vi "NonDuplicateArrays.vi"(8 "error in":errorcluster, 9 "string in":string, 11 "array in":string[](array[string])) -> (0 "error out":errorcluster, 3 "array out":string[](array[string]))   [LabVIEW 2023, in "CEF.lvlib"]
doc: "This Vi checks if the string exist in the array, if it doesnt it adds it to the array.Copyright 2017 National Instruments Corporation\n\nLicensed under the Apache License, Version 2.0 (the \"License\"); you may not use this file except in compliance with the License. You may obtain a copy of the License at http://www.apache.org/licenses/LICENSE-2.0\nUnless required by applicable law or agreed to in writing, software distributed under the License is distributed on an \"AS IS\" BASIS, WITHOUT WARRANTIES OR CONDITIONS OF ANY KIND, either express or implied. See the License for the specific language governing permissions and limitations under the License."
uses:
  CEF.lvlib
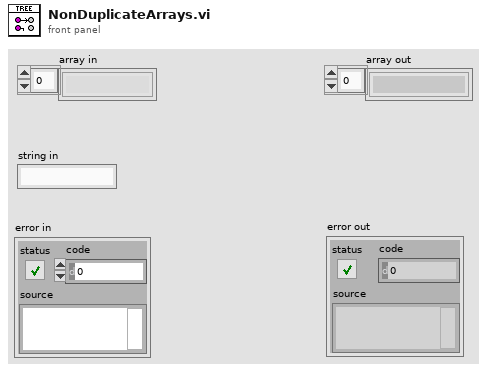
[diagram p1: front panel]
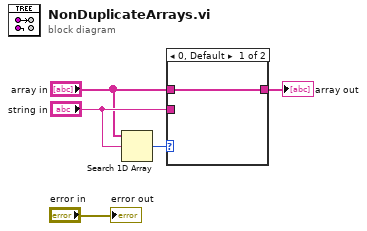
[diagram p0: block diagram]
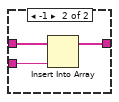
[diagram p2: hidden frame]
diagram:
  n1 = Search 1D Array(1D array="array in", element="string in") -> (index of element=w1:i32)  [unwired: 1 in]
  n2 = case shown="0, Default" w1 {
    tunnel: [w6 w8] -> w2
    tunnel: "array in" -> [w6 w9]
    tunnel: "string in" -> [_ w7]
    frame 0, Default {
    }
    frame -1 {
      n3 = Insert Into Array(array=w9, new element=w7) -> (w8:string[])  [unwired: 1 in]
    }
  }
  "array out" <- w2
  "error out" <- "error in"
